vi "Main - Separate File and Output sessions.vi"() -> ()   [LabVIEW 2012]
uses:
  ChannelStateControl.ctl
  Imaging Pulse Control/Examples/Support/Channel Parameters.ctl
  Imaging Pulse Control/Examples/Support/System Parameters.ctl
  <vilib>/UeiDaq/UeiDaqCreateDOSession.vi
  <vilib>/UeiDaq/UeiDaqConfigureTimingForSimpleIO.vi
  <vilib>/UeiDaq/UeiDaqWriteDigitalDataUInt16.vi
  <vilib>/UeiDaq/UeiDaqWriteOneDigitalScanUInt16.vi
  <resource>/objmgr/UeiDaq.rc
  <vilib>/Utility/error.llb/DialogType.ctl
  <vilib>/ULx/Write.llb/ULx Write (Analog 1D DBL NChan 1Samp).vi
  Imaging Pulse Control/Quantum Composers 9000 Series.lvlib
  <vilib>/ULx/Create Channel.llb/ULx Create Channel (AO-Voltage-Basic).vi
  IPG Pulse Control/Agilent 33XXX Series.lvlib
  Agilent ESG Series/Agilent ESG Series.lvlib
panel:
  out "Timing Changed?":bool
  in  "Generate Form Switch":bool
  out "Period":dbl
  in  "#DIO Ports (Adjustable)":i32
  in  "Composer Write":bool
  in  "VISA session":refnum<visa-resource-name>
  in  "error in (no error)":errorcluster {"code" format="%.0x"}
  out "error out":errorcluster {"code" format="%.0x"}
  in  "Frequency (MHz)":dbl=224.0 format="%.11f"
  in  "Amplitude (dBm)":dbl=7.0 format="%.2f"
  in  "Output Enable":bool=TRUE
  out "Offset":dbl
  out "Amplitude":dbl
  in  "Maximum Voltage":dbl=10.0
  in  "Initial Voltage":dbl=2.0
  in  "Final Voltage":dbl=4.0
  out "Frequency":dbl=0.4838
  in  "Trigger Source (0: Internal)":u16(ring)=1 items=["Internal", "External", "Software (bus)"]
  in  "Enable Burst":bool=TRUE
  in  "Burst Mode (0: Triggered)":u16(ring) items=["Triggered", "Gated"]
  out "Simulated WaveForm":dbl[](graph)
  out "Total Time  (<16000)":i32
  in  "Final Keep Time":i32=100
  in  "Fall Down Time":i32=1000
  in  "Rise Up Time":i32=15
  in  "Pulse Width":i32=100
  in  "Inintial Voltage Time":i32=1
  in  "IPG Controller (Agilent 33210A)":refnum<visa-resource-name>
  in  "Arbitrary Waveform Name":string="ARB1"
  in  "Run IPG Laser  Switch":bool
  in  "Normal Stop":bool
  in  "Voltage (V)":dbl[](array[numeric])
  out "Initial States":u16[](array[numeric])
  in  "DIO Groups":T1[](array[typedef])=[{"Channel 1"=0, "Enable"=TRUE, "Main Switch"=0, "Channel 2"=0, "Channel 9"=0, "Channel 10"=0, "Channel 11"=0, "Channel 3"=0, "Channel 4"=0, "Channel 12"=0, "Channel 5"=0, "Channel 13"=0, "Channel 6"=0, "Channel 14"=0, "Channel 7"=0, "Channel 15"=0, "Channel 8"=0, "Channel 16"=0}, {"Channel 1"=0, "Enable"=TRUE, "Main Switch"=0, "Channel 2"=0, "Channel 9"=0, "Channel 10"=0, "Channel 11"=0, "Channel 3"=0, "Channel 4"=0, "Channel 12"=0, "Channel 5"=0, "Channel 13"=0, "Channel 6"=0, "Channel 14"=0, "Channel 7"=0, "Channel 15"=0, "Channel 8"=0, "Channel 16"=0}, {"Channel 1"=0, "Enable"=TRUE, "Main Switch"=0, "Channel 2"=0, "Channel 9"=0, "Channel 10"=0, "Channel 11"=0, "Channel 3"=0, "Channel 4"=0, "Channel 12"=0, "Channel 5"=0, "Channel 13"=0, "Channel 6"=0, "Channel 14"=0, "Channel 7"=0, "Channel 15"=0, "Channel 8"=0, "Channel 16"=0}, {"Channel 1"=0, "Enable"=TRUE, "Main Switch"=0, "Channel 2"=0, "Channel 9"=0, "Channel 10"=0, "Channel 11"=0, "Channel 3"=0, "Channel 4"=0, "Channel 12"=0, "Channel 5"=0, "Channel 13"=0, "Channel 6"=0, "Channel 14"=0, "Channel 7"=0, "Channel 15"=0, "Channel 8"=0, "Channel 16"=0}, {"Channel 1"=0, "Enable"=TRUE, "Main Switch"=0, "Channel 2"=0, "Channel 9"=0, "Channel 10"=0, "Channel 11"=0, "Channel 3"=0, "Channel 4"=0, "Channel 12"=0, "Channel 5"=0, "Channel 13"=0, "Channel 6"=0, "Channel 14"=0, "Channel 7"=0, "Channel 15"=0, "Channel 8"=0, "Channel 16"=0}, {"Channel 1"=0, "Enable"=TRUE, "Main Switch"=0, "Channel 2"=0, "Channel 9"=0, "Channel 10"=0, "Channel 11"=0, "Channel 3"=0, "Channel 4"=0, "Channel 12"=0, "Channel 5"=0, "Channel 13"=0, "Channel 6"=0, "Channel 14"=0, "Channel 7"=0, "Channel 15"=0, "Channel 8"=0, "Channel 16"=0}]
  out "Quantum Composer Command":string[](array[string])
  in  "Sys Period (s)":dbl=0.15
  out "Composer Ready?":bool
  out "Main Loop Stopped?":bool
  in  "Quantum Composer Resource":refnum<visa-resource-name>
  in  "Run/Stop":bool caption="stop"
  in  "Exit":bool
  out "Running 2":bool
  in  "Maximum Value":dbl=5.5 format="%0.2f"
  in  "Minimum Value":dbl format="%0.2f"
  out "Status Indicator":bool[][](array[boolean])
  out "Total Step":u64
  out "Original Timing Signal":i16[][](array[numeric]) format="%b"
  out "Running":bool
  in  "DIO Port":string="pwrdaq://Dev0/Do0:2"
  in  "stop":bool
  out "Loop Count":i32
  in  "Loop":bool
  out "Parsed File Location":path
  in  "All Low":bool
  in  "Run":bool
  in  "Timing Array (Adjustable)":i32[](array[numeric])=[0, 0, 0, 0, 0, 0, 0, 0, 0, 0, 0, 0, 0, 0, 0, 0, 0, 0, 0, 0] caption="Timing Array (Time Duration for each signal)"
  in  "Modified Timing Signal":i16[][](array[numeric])=[[0, 0, 0, 0, 0, 0, 0, 0, 0, 0, 0, 0, 0, 0, 0, 0, 0, 0, 0, 0]] caption="Modified Timing Signal (after adjustment from I/O channel panel)" format="%b"
  in  "Compile and Load":bool
  out "Channel Names":string[](array[string])
  out "Channel Number":u16=48
  in  "Timing File":path
  in  "Perl Parser":path=path "C:/Labview/Parser File/parse-timing.pl"
  # "MCCDAQ Control"
  # "Quantum Composer Control"
  # "(Use Do0:5 for DIO0-DIO5, 6ch,  Do0;5 for DIO0 and DIO5, 2ch)"
  # "Control Panel"
  # "(pwrdaq://Dev0 for real I/O; simu://Dev2 for simulated DAQ card)"
  # "1"
  # "2"
  # "3"
  # "4"
  # "5"
  # "6"
  # "7"
  # "8"
  # "9"
  # "10"
  # "11"
  # "12"
  # "13"
  # "14"
  # "15"
  # "16"
  # "Read me: (Very Important!!!!!!!!!)\n1. This Labview is used to control the IPG laser output power, When you edit this programme make sure the IPG laser is off.\n2. follow the steps, First is the visa address setting; Second is the pulse edit; Third is the output checking; Forth is the trigger set .\n3. The maximum input voltage is 10V, the minmum value is 1V. The total input time must smaller than 16000ms and larger than 8 ms."
  # "Group1"
  # "Group2"
  # "Group3"
  # "IPG Modulation Control"
  # "Offset Locking Control"
  # "Group4"
  # "Group5"
  # "Group6"
  # "(Currently, When \"STOP Loop\" is pressed, the status remain in the final state, when Stop Program or ER stop is pressed, all channels will be set as \"low\")"
  # "Status Panel"
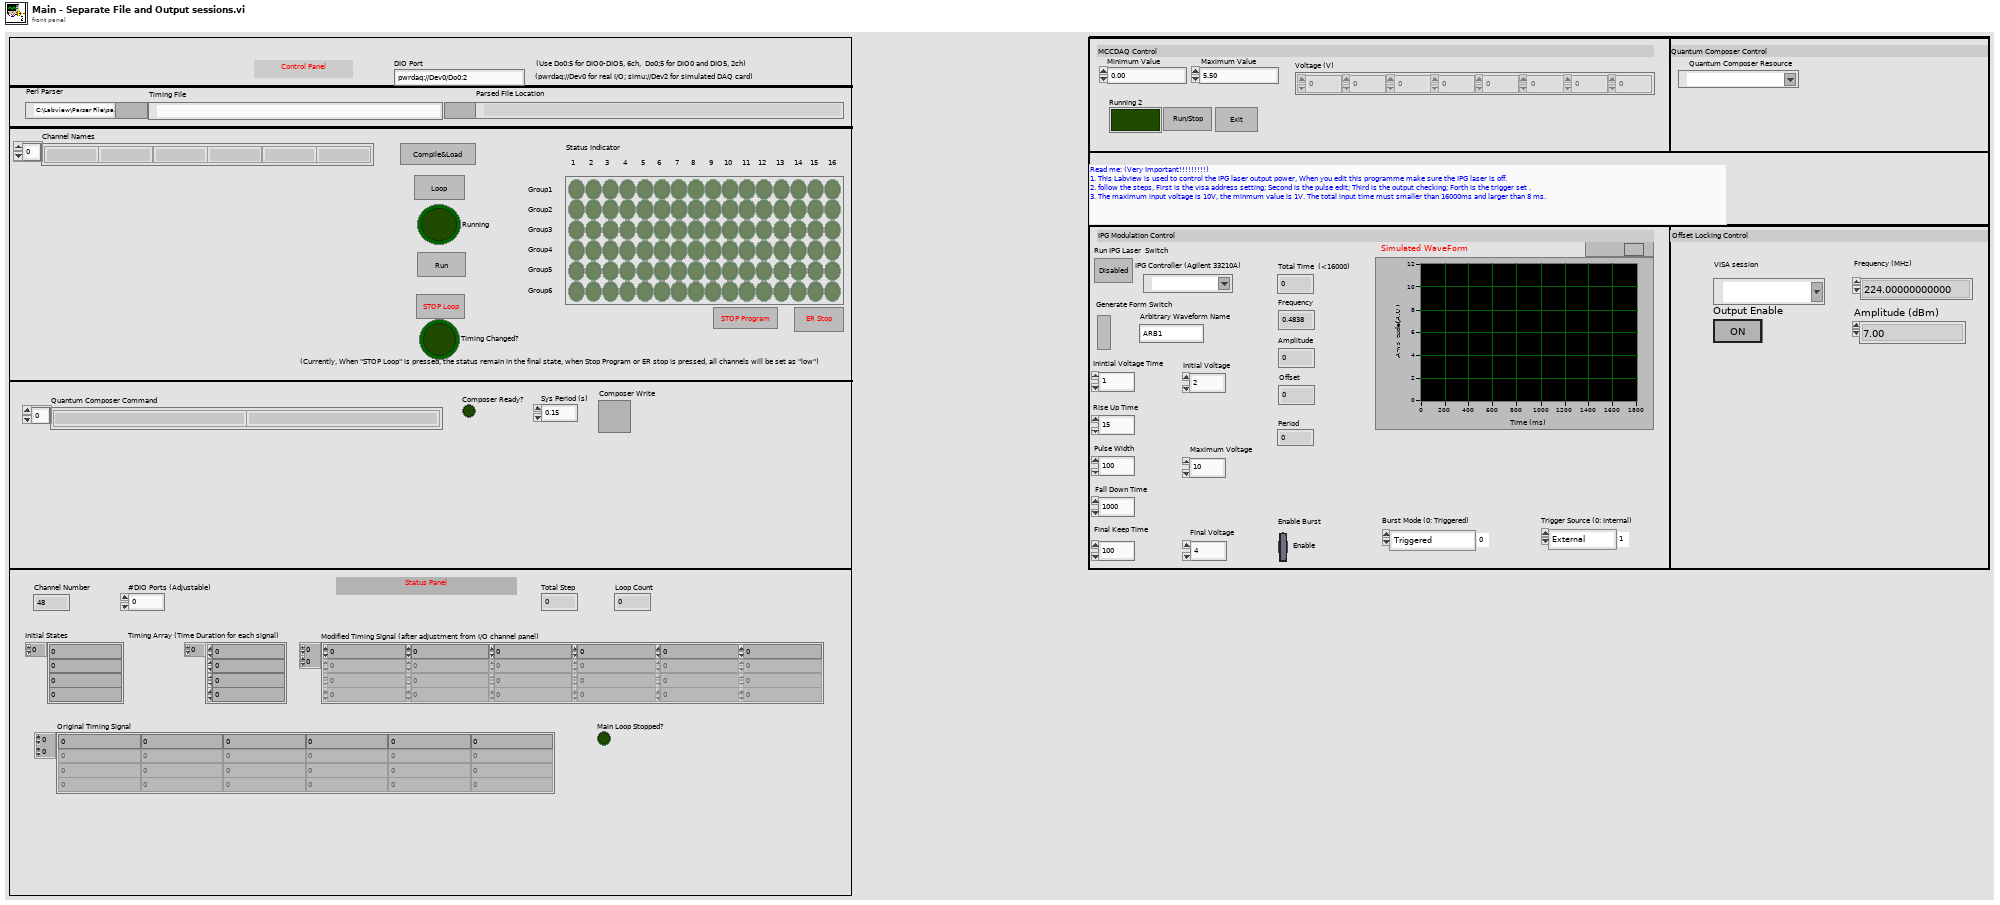
[diagram p1: front panel]
types:
  T1 = typedef "ChannelStateControl.ctl" = cluster{"Channel 1":u8, "Enable":bool, "Main Switch":u8, "Channel 2":u8, "Channel 9":u8, "Channel 10":u8, "Channel 11":u8, "Channel 3":u8, "Channel 4":u8, "Channel 12":u8, "Channel 5":u8, "Channel 13":u8, "Channel 6":u8, "Channel 14":u8, "Channel 7":u8, "Channel 15":u8, "Channel 8":u8, "Channel 16":u8}
  T2 = typedef "Channel Parameters.ctl" = cluster{"Channel":i32, "Chan State":bool, "Chan Sync Source":i32, "Chan Gate Logic":enum16{"Disabled", "Low", "High"}, "Chan Mode":enum16{"Normal", "Single", "Burst", "Duty Cycle"}, "Chan Wait #":i32, "Chan Delay":dbl, "Chan Width":dbl, "Chan Burst #":i32, "Chan DC On":i32, "Chan DC Off":i32, "Chan Polarity":bool, "Chan MUX Value":i32, "Chan Level Out":enum16{"TTL", "Adjustable", "35 Volt", "Optical"}, "Chan Lev Adjust":dbl, "Chan Gate Mode":enum16{"Disabled", "Pulse Inhibit", "Output Inhibit"}}
  T3 = enum16{"dBm", "dBuV", "dBuVemf", "mV", "uV", "mVemf", "uVemf"}
  T4 = enum16{"SINE", "TRIANGLE", "SQUARE", "RAMP", "NOISE", "DUAL SINE", "SWEPT SINE"}
  T5 = typedef "DialogType.ctl" = u16
  T6 = typedef "System Parameters.ctl" = cluster{"Sys Period":dbl, "Sys Mode":enum16{"Normal", "Single", "Burst", "Duty Cycle"}, "Sys Burst #":i32, "Sys DC On":i32, "Sys DC Off":i32, "Sys State":bool, "Sys Gate":bool, "Sys Trig Edge":bool, "Sys Ext Mode":enum16{"Disabled", "Triggered", "Gated", "Triggered & Gated"}, "Sys Trig Lev":dbl, "Sys Gate Lev ":dbl, "Sys Gate Mode":enum16{"Disabled", "Pulse Inhibit", "Output Inhibit", "Channel"}}
  T7 = cluster{"Baud Rate":u32, "Parity":u16, "Data Bits":u16, "Flow Control":u16}
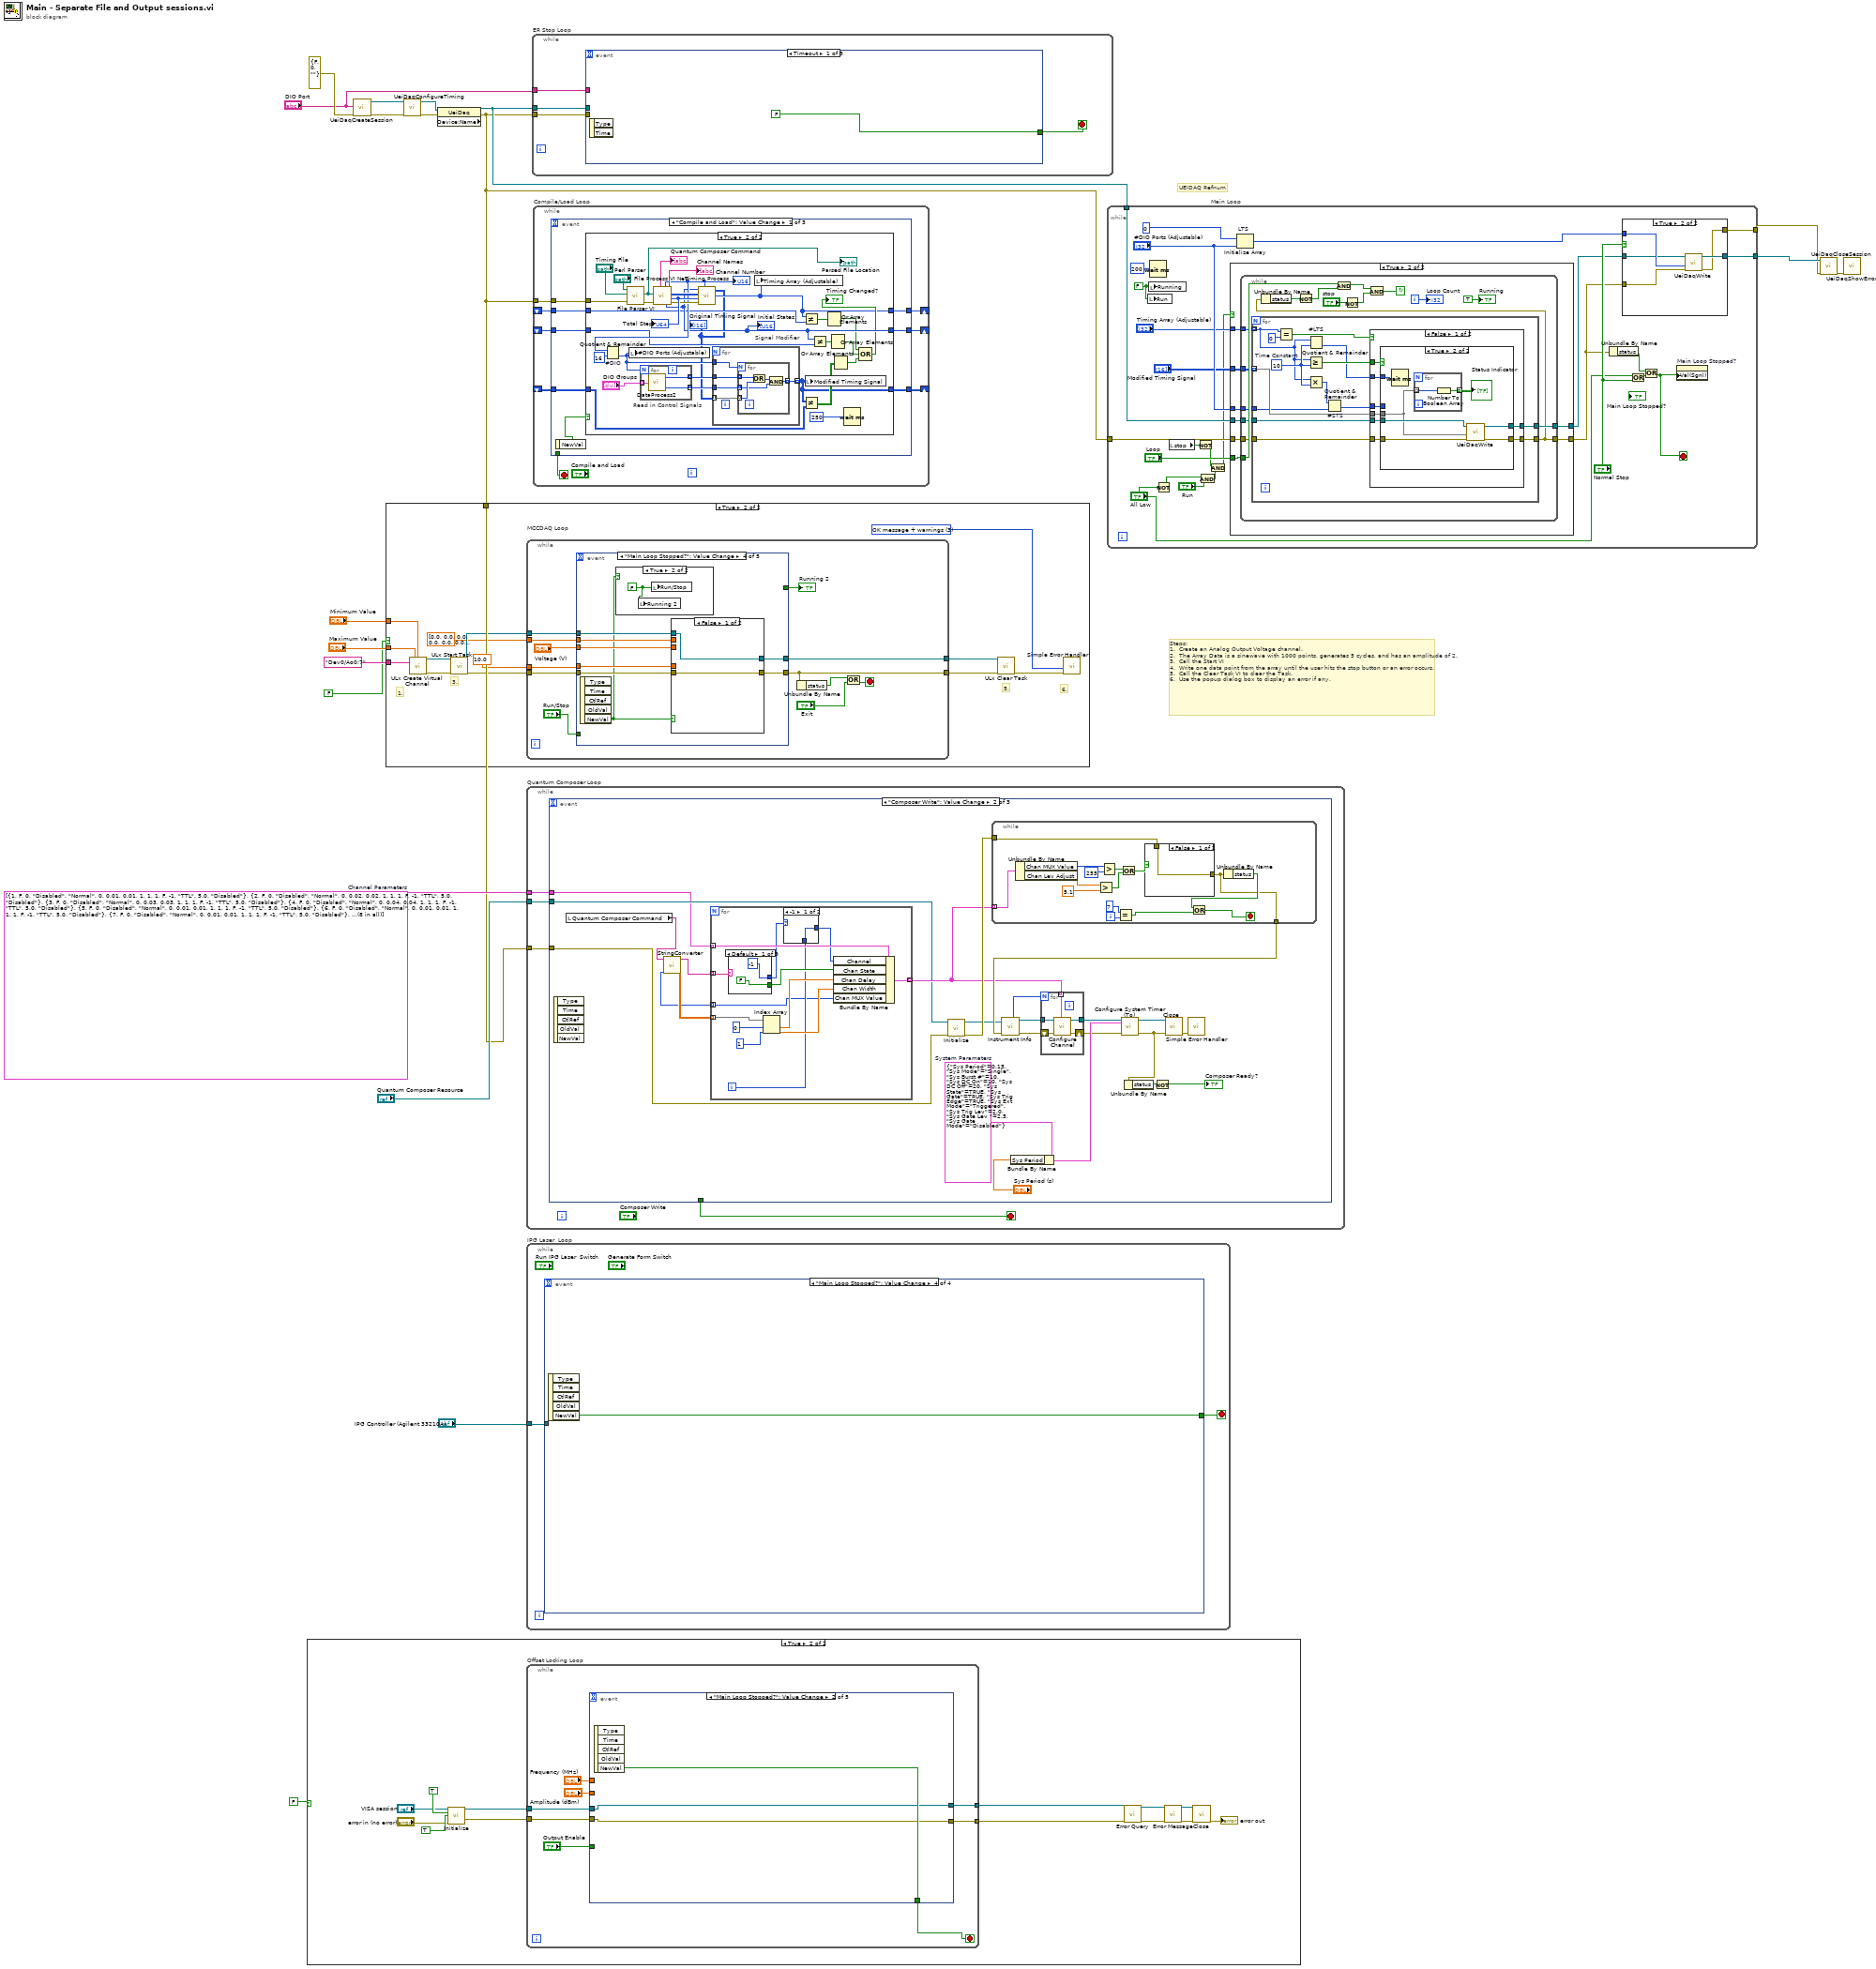
[diagram p0: block diagram]
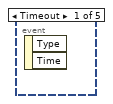
[diagram p3: hidden frame]
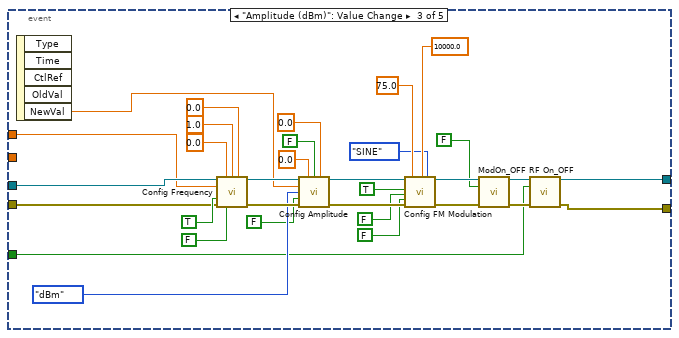
[diagram p4: hidden frame]
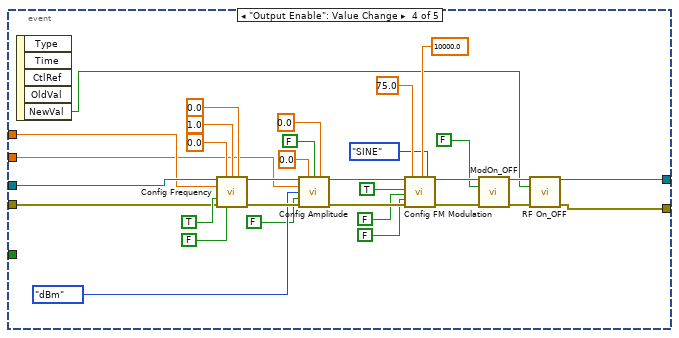
[diagram p5: hidden frame]
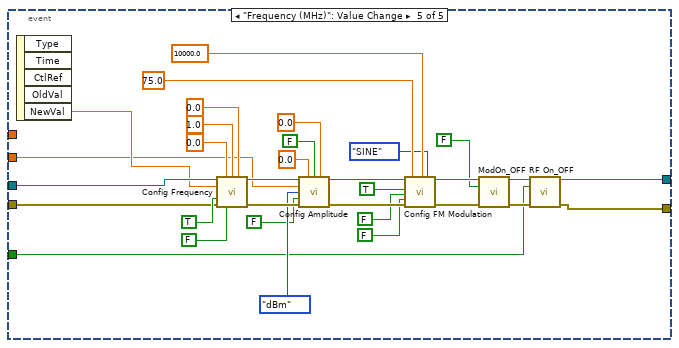
[diagram p6: hidden frame]
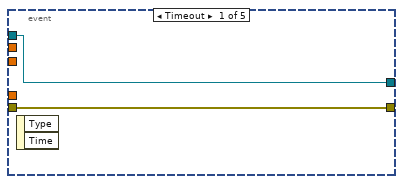
[diagram p8: hidden frame]
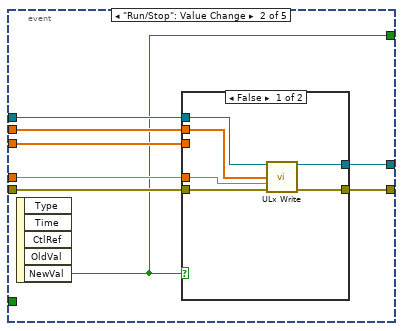
[diagram p9: hidden frame]
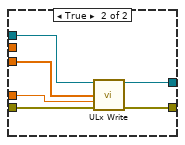
[diagram p10: hidden frame]
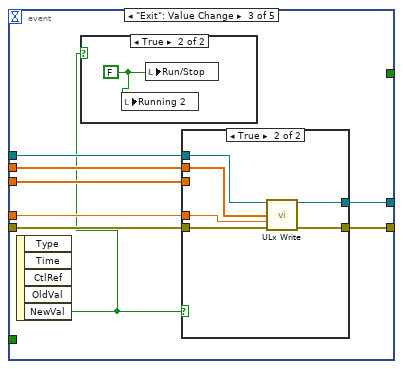
[diagram p11: hidden frame]
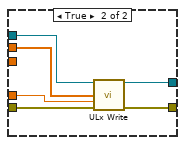
[diagram p15: hidden frame]
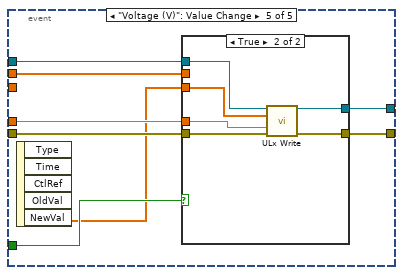
[diagram p16: hidden frame]
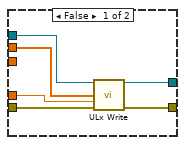
[diagram p17: hidden frame]
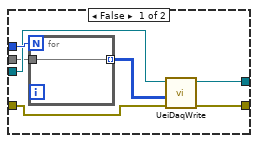
[diagram p20: hidden frame]
diagram:
  w8 = T2[] [{"Channel"=1, "Chan State"=FALSE, "Chan Sync Source"=0, "Chan Gate Logic"=enum."Disabled", "Chan Mode"=enum."Normal", "Chan Wait #"=0, "Chan Delay"=0.01, "Chan Width"=0.01, "Chan Burst #"=1, "Chan DC On"=1, "Chan DC Off"=1, "Chan Polarity"=FALSE, "Chan MUX Value"=-1, "Chan Level Out"=enum."TTL", "Chan Lev Adjust"=5.0, "Chan Gate Mode"=enum."Disabled"}, {"Channel"=2, "Chan State"=FALSE, "Chan Sync Source"=0, "Chan Gate Logic"=enum."Disabled", "Chan Mode"=enum."Normal", "Chan Wait #"=0, "Chan Delay"=0.02, "Chan Width"=0.02, "Chan Burst #"=1, "Chan DC On"=1, "Chan DC Off"=1, "Chan Polarity"=FALSE, "Chan MUX Value"=-1, "Chan Level Out"=enum."TTL", "Chan Lev Adjust"=5.0, "Chan Gate Mode"=enum."Disabled"}, {"Channel"=3, "Chan State"=FALSE, "Chan Sync Source"=0, "Chan Gate Logic"=enum."Disabled", "Chan Mode"=enum."Normal", "Chan Wait #"=0, "Chan Delay"=0.03, "Chan Width"=0.03, "Chan Burst #"=1, "Chan DC On"=1, "Chan DC Off"=1, "Chan Polarity"=FALSE, "Chan MUX Value"=-1, "Chan Level Out"=enum."TTL", "Chan Lev Adjust"=5.0, "Chan Gate Mode"=enum."Disabled"}, {"Channel"=4, "Chan State"=FALSE, "Chan Sync Source"=0, "Chan Gate Logic"=enum."Disabled", "Chan Mode"=enum."Normal", "Chan Wait #"=0, "Chan Delay"=0.04, "Chan Width"=0.04, "Chan Burst #"=1, "Chan DC On"=1, "Chan DC Off"=1, "Chan Polarity"=FALSE, "Chan MUX Value"=-1, "Chan Level Out"=enum."TTL", "Chan Lev Adjust"=5.0, "Chan Gate Mode"=enum."Disabled"}, {"Channel"=5, "Chan State"=FALSE, "Chan Sync Source"=0, "Chan Gate Logic"=enum."Disabled", "Chan Mode"=enum."Normal", "Chan Wait #"=0, "Chan Delay"=0.01, "Chan Width"=0.01, "Chan Burst #"=1, "Chan DC On"=1, "Chan DC Off"=1, "Chan Polarity"=FALSE, "Chan MUX Value"=-1, "Chan Level Out"=enum."TTL", "Chan Lev Adjust"=5.0, "Chan Gate Mode"=enum."Disabled"}, {"Channel"=6, "Chan State"=FALSE, "Chan Sync Source"=0, "Chan Gate Logic"=enum."Disabled", "Chan Mode"=enum."Normal", "Chan Wait #"=0, "Chan Delay"=0.01, "Chan Width"=0.01, "Chan Burst #"=1, "Chan DC On"=1, "Chan DC Off"=1, "Chan Polarity"=FALSE, "Chan MUX Value"=-1, "Chan Level Out"=enum."TTL", "Chan Lev Adjust"=5.0, "Chan Gate Mode"=enum."Disabled"}, {"Channel"=7, "Chan State"=FALSE, "Chan Sync Source"=0, "Chan Gate Logic"=enum."Disabled", "Chan Mode"=enum."Normal", "Chan Wait #"=0, "Chan Delay"=0.01, "Chan Width"=0.01, "Chan Burst #"=1, "Chan DC On"=1, "Chan DC Off"=1, "Chan Polarity"=FALSE, "Chan MUX Value"=-1, "Chan Level Out"=enum."TTL", "Chan Lev Adjust"=5.0, "Chan Gate Mode"=enum."Disabled"}, {"Channel"=8, "Chan State"=FALSE, "Chan Sync Source"=0, "Chan Gate Logic"=enum."Disabled", "Chan Mode"=enum."Normal", "Chan Wait #"=0, "Chan Delay"=0.01, "Chan Width"=0.01, "Chan Burst #"=1, "Chan DC On"=1, "Chan DC Off"=1, "Chan Polarity"=FALSE, "Chan MUX Value"=-1, "Chan Level Out"=enum."TTL", "Chan Lev Adjust"=5.0, "Chan Gate Mode"=enum."Disabled"}]  # Channel Parameters
  # "UEIDAQ Refnum"
  # "Steps: \n1.  Create an Analog Output Voltage channel.\n2.  The Array Data is a sinewave with 1000 points, generates 5 cycles, and has an amplitude of 2.\n3.  Call the Start VI\n4.  Write one data point from the array until the user hits the stop button or an error occurs. \n5.  Call the Clear Task VI to clear the Task.\n6.  Use the popup dialog box to display an error if any."
  n1 = case shown="True" FALSE {
    frame False {
    }
    frame True {
      n2 = call "Initialize.vi"("VISA Resource Name"="VISA session", "ID Query? (T: Yes)"=TRUE, "Reset? (T: Yes)"=TRUE, "error in (no error)"="error in (no error)") -> ("VISA Resource Name Out"=w22:refnum<visa-resource-name>, "error out"=w21:errorcluster)  [unwired: 10 in]
      n3 = while "Offset Locking Loop" {
        tunnel: [w40] -> w27
        tunnel: w22 -> [w39]
        tunnel: w21 -> [w38]
        tunnel: [w37] -> w20
        stop <- w35 stop-if-true
        n4 = event shown="[1] \"Main Loop Stopped?\": Value Change" {
          selector: _ -> [_ _ _ _ _]
          dyn-events: _ -> [_ _ _ _ _]
          timeout: _ -> [_ _ _ _ _]
          tunnel: [_ w41 w50 w82 w114] -> w40
          tunnel: w39 -> [_ w42 w49 w81 w113]
          tunnel: w38 -> [_ w41 w48 w80 w112]
          tunnel: "Output Enable" -> [_ _ w47 _ w109]
          tunnel: [_ w42 w46 w79 w108] -> w37
          tunnel: "Frequency (MHz)" -> [_ _ w44 w78 _]
          tunnel: [_ w43 _ _ _] -> w35
          tunnel: "Amplitude (dBm)" -> [_ _ _ w77 w110]
          event Timeout {
            n5 = event-data() -> ()  [unwired: 1 in, 2 out]
          }
          event "Main Loop Stopped?": Value Change {
            n6 = event-data() -> ("NewVal"=w43:bool)  [unwired: 1 in, 4 out]
          }
          event "Amplitude (dBm)": Value Change {
            n7 = event-data() -> ("NewVal"=w45:dbl)  [unwired: 1 in, 4 out]
            n8 = call "Config Frequency.vi"("VISA Resource Name"=w49, "Freq Offset (0.0)"=0.0, "Freq Multiplier (1.0)"=1.0, "Adjust Phase (0.0)"=0.0, "Frequency (1000.0)"=w44, "Freq Ref (T:ON)"=TRUE, "error in (no error)"=w48, "OptPhNoise (F:MD2 > 10khzOffset)"=FALSE) -> ("VISA Resource Name Out"=w75:refnum<visa-resource-name>, "error out"=w74:errorcluster)  [unwired: 6 in]
            n9 = call "Config Amplitude.vi"("VISA Resource Name"=w75, "Ampl Ref Set (0.00)"=0.0, "Ampl Ref (F:OFF)"=FALSE, "Ampl Offset (0.00)"=0.0, "Amplitude (-135.00)"=w45, "Unit (0:dBm)"=T3."dBm", "Atten Hold (F:OFF)"=FALSE, "error in (no error)"=w74) -> ("VISA Resource Name Out"=w73:refnum<visa-resource-name>, "error out"=w72:errorcluster)  [unwired: 6 in]
            n10 = call "Config FM Modulation.vi"("VISA Resource Name"=w73, "Status (T:ON)"=TRUE, "EXT Source Coupling (F:DC)"=FALSE, "FM Deviation Couple (F:OFF)"=FALSE, "error in (no error)"=w72, "FM Deviation (1.0)"=75.0 ("FM Deviation (75)"), "FM Rate (400.0)"=10000.0 ("FM Rate (10000)"), "FM Waveform (0:SINE)"=T4."SINE") -> ("VISA Resource Name Out"=w71:refnum<visa-resource-name>, "error out"=w70:errorcluster)  [unwired: 10 in]
            n11 = call "ModOn_OFF.vi"("VISA Resource Name"=w71, "Status (T:ON)"=FALSE, "error in (no error)"=w70) -> ("VISA Resource Name Out"=w69:refnum<visa-resource-name>, "error out"=w68:errorcluster)  [unwired: 11 in]
            n12 = call "RF On_OFF.vi"("VISA Resource Name"=w69, "Status (T:ON)"=w47, "error in (no error)"=w68) -> ("VISA Resource Name Out"=w46:refnum<visa-resource-name>, "error out"=w50:errorcluster)  [unwired: 11 in]
          }
          event "Output Enable": Value Change {
            n13 = event-data() -> ("NewVal"=w76:bool)  [unwired: 1 in, 4 out]
            n14 = call "Config Frequency.vi"("VISA Resource Name"=w81, "Freq Offset (0.0)"=0.0, "Freq Multiplier (1.0)"=1.0, "Adjust Phase (0.0)"=0.0, "Frequency (1000.0)"=w78, "Freq Ref (T:ON)"=TRUE, "error in (no error)"=w80, "OptPhNoise (F:MD2 > 10khzOffset)"=FALSE) -> ("VISA Resource Name Out"=w107:refnum<visa-resource-name>, "error out"=w106:errorcluster)  [unwired: 6 in]
            n15 = call "Config Amplitude.vi"("VISA Resource Name"=w107, "Ampl Ref Set (0.00)"=0.0, "Ampl Ref (F:OFF)"=FALSE, "Ampl Offset (0.00)"=0.0, "Amplitude (-135.00)"=w77, "Unit (0:dBm)"=T3."dBm", "Atten Hold (F:OFF)"=FALSE, "error in (no error)"=w106) -> ("VISA Resource Name Out"=w105:refnum<visa-resource-name>, "error out"=w104:errorcluster)  [unwired: 6 in]
            n16 = call "Config FM Modulation.vi"("VISA Resource Name"=w105, "Status (T:ON)"=TRUE, "EXT Source Coupling (F:DC)"=FALSE, "FM Deviation Couple (F:OFF)"=FALSE, "error in (no error)"=w104, "FM Deviation (1.0)"=75.0 ("FM Deviation (75)"), "FM Rate (400.0)"=10000.0 ("FM Rate (10000)"), "FM Waveform (0:SINE)"=T4."SINE") -> ("VISA Resource Name Out"=w103:refnum<visa-resource-name>, "error out"=w102:errorcluster)  [unwired: 10 in]
            n17 = call "ModOn_OFF.vi"("VISA Resource Name"=w103, "Status (T:ON)"=FALSE, "error in (no error)"=w102) -> ("VISA Resource Name Out"=w101:refnum<visa-resource-name>, "error out"=w100:errorcluster)  [unwired: 11 in]
            n18 = call "RF On_OFF.vi"("VISA Resource Name"=w101, "Status (T:ON)"=w76, "error in (no error)"=w100) -> ("VISA Resource Name Out"=w79:refnum<visa-resource-name>, "error out"=w82:errorcluster)  [unwired: 11 in]
          }
          event "Frequency (MHz)": Value Change {
            n19 = event-data() -> ("NewVal"=w111:dbl)  [unwired: 1 in, 4 out]
            n20 = call "Config Frequency.vi"("VISA Resource Name"=w113, "Freq Offset (0.0)"=0.0, "Freq Multiplier (1.0)"=1.0, "Adjust Phase (0.0)"=0.0, "Frequency (1000.0)"=w111, "Freq Ref (T:ON)"=TRUE, "error in (no error)"=w112, "OptPhNoise (F:MD2 > 10khzOffset)"=FALSE) -> ("VISA Resource Name Out"=w139:refnum<visa-resource-name>, "error out"=w138:errorcluster)  [unwired: 6 in]
            n21 = call "Config Amplitude.vi"("VISA Resource Name"=w139, "Ampl Ref Set (0.00)"=0.0, "Ampl Ref (F:OFF)"=FALSE, "Ampl Offset (0.00)"=0.0, "Amplitude (-135.00)"=w110, "Unit (0:dBm)"=T3."dBm", "Atten Hold (F:OFF)"=FALSE, "error in (no error)"=w138) -> ("VISA Resource Name Out"=w137:refnum<visa-resource-name>, "error out"=w136:errorcluster)  [unwired: 6 in]
            n22 = call "Config FM Modulation.vi"("VISA Resource Name"=w137, "Status (T:ON)"=TRUE, "EXT Source Coupling (F:DC)"=FALSE, "FM Deviation Couple (F:OFF)"=FALSE, "error in (no error)"=w136, "FM Deviation (1.0)"=75.0 ("FM Deviation (75)"), "FM Rate (400.0)"=10000.0 ("FM Rate (10000)"), "FM Waveform (0:SINE)"=T4."SINE") -> ("VISA Resource Name Out"=w135:refnum<visa-resource-name>, "error out"=w134:errorcluster)  [unwired: 10 in]
            n23 = call "ModOn_OFF.vi"("VISA Resource Name"=w135, "Status (T:ON)"=FALSE, "error in (no error)"=w134) -> ("VISA Resource Name Out"=w133:refnum<visa-resource-name>, "error out"=w132:errorcluster)  [unwired: 11 in]
            n24 = call "RF On_OFF.vi"("VISA Resource Name"=w133, "Status (T:ON)"=w109, "error in (no error)"=w132) -> ("VISA Resource Name Out"=w108:refnum<visa-resource-name>, "error out"=w114:errorcluster)  [unwired: 11 in]
          }
        }
      }
      n25 = call "Error Query.vi"("VISA Resource Name"=w20, "error in (no error)"=w27) -> ("VISA Resource Name Out"=w29:refnum<visa-resource-name>, "error out"=w32:errorcluster)  [unwired: 10 in, 2 out]
      n26 = call "Error Message.vi"("VISA Resource Name"=w29, "error in (no error)"=w32) -> ("VISA Resource Name Out"=w30:refnum<visa-resource-name>, "error out"=w31:errorcluster)  [unwired: 9 in, 3 out]
      n27 = call "Close.vi"("VISA Resource Name"=w30, "error in (no error)"=w31) -> ("error out"=→"error out":errorcluster)  [unwired: 13 in]
    }
  }
  n28 = call-poly <vilib>:"UeiDaqCreateSession.vi"("error in (no error)"=errorcluster {"status"=FALSE, "code"=0, "source"=""} ("error constant"), "Resource"="DIO Port") -> ("error out"=w18:errorcluster, "UeiDaq Refnum Out"=w19:refnum<k20>)  [unwired: 8 in]
  n29 = call-poly <vilib>:"UeiDaqConfigureTiming.vi"("error in (no error)"=w18, "UeiDaq Refnum In"=w19) -> ("error out"=w16:errorcluster, "UeiDaq Refnum Out"=w17:refnum<k20>)  [unwired: 8 in]
  n30 = property class="UeiDaq" props=["Device:Name"](reference=w17, error in=w16) -> (reference out=w7:refnum<k20>, error out=w6:errorcluster)  [unwired: 1 out]
  n31 = case shown="True" FALSE {
    tunnel: "Minimum Value" -> [_ w153]
    tunnel: "Maximum Value" -> [_ w152]
    tunnel: "Dev0/Ao0:7" -> [_ w145]
    tunnel: w6 -> [_ w140]
    frame False {
    }
    frame True {
      w148 = T5 3 items=["no dialog", "OK message", "continue or stop message", "OK message + warnings", "continue/stop + warnings"] ("type of dialog (OK msg:1)")
      # "6."
      # "5."
      # "3."
      # "1."
      n32 = call-poly <vilib>:"ULx Create Virtual Channel.vi"("maximum value"=w152, "minimum value"=w153, "physical channels"=w145, "error in"=w140) -> ("task out"=w147:refnum<k24>, "error out"=w146:errorcluster)  [unwired: 10 in]
      n33 = call <vilib>:"ULx Start Task.vi"("task in"=w147, "error in"=w146) -> ("task out"=w149:refnum<k24>, "error out"=w151:errorcluster)  [unwired: 12 in]
      n34 = while "MCCDAQ Loop" {
        tunnel: w151 -> [w164]
        tunnel: w149 -> [w165]
        tunnel: dbl[] [0.0, 0.0, 0.0, 0.0, 0.0, 0.0, 0.0, 0.0] -> [w161]
        tunnel: [w163] -> w144
        tunnel: [w160] -> w143
        tunnel: 10.0 ("timeout") -> [w162]
        stop <- w159 stop-if-true
        n35 = event shown="[3] \"Main Loop Stopped?\": Value Change" {
          selector: _ -> [_ _ _ _ _]
          dyn-events: _ -> [_ _ _ _ _]
          timeout: _ -> [_ _ _ _ _]
          tunnel: w165 -> [w167 w175 w195 w212 w229]
          tunnel: w164 -> [w166 w174 w194 w211 w228]
          tunnel: w162 -> [_ w173 w193 w210 w227]
          tunnel: "Voltage (V)" -> [_ w172 w192 w209 _]
          tunnel: [w167 w171 w191 w208 w226] -> w163
          tunnel: [w166 w170 w190 w207 w225] -> w160
          tunnel: w161 -> [_ w169 w189 w206 w224]
          tunnel: "Run/Stop" -> [_ _ _ _ w223]
          tunnel: [_ w168 _ _ _] -> w155
          event Timeout {
            n36 = event-data() -> ()  [unwired: 1 in, 2 out]
          }
          event "Run/Stop": Value Change {
            n37 = event-data() -> ("NewVal"=w168:bool)  [unwired: 1 in, 4 out]
            n38 = case shown="False" w168 {
              tunnel: w175 -> [w179 w187]
              tunnel: w174 -> [w178 w186]
              tunnel: w173 -> [w180 w185]
              tunnel: w172 -> [_ w184]
              tunnel: [w177 w183] -> w171
              tunnel: [w176 w182] -> w170
              tunnel: w169 -> [w181 _]
              frame False {
                n39 = call-poly <vilib>:"ULx Write.vi"("task in"=w179, "data"=w181, "timeout"=w180, "error in"=w178) -> ("task out"=w177:refnum<k24>, "error out"=w176:errorcluster)  [unwired: 9 in, 1 out]
              }
              frame True {
                n40 = call-poly <vilib>:"ULx Write.vi"("task in"=w187, "data"=w184, "timeout"=w185, "error in"=w186) -> ("task out"=w183:refnum<k24>, "error out"=w182:errorcluster)  [unwired: 9 in, 1 out]
              }
            }
          }
          event "Exit": Value Change {
            n41 = event-data() -> ("NewVal"=w188:bool)  [unwired: 1 in, 4 out]
            n42 = case shown="True" w188 {
              frame False {
              }
              frame True {
                w196 = FALSE
                n43 = local write "Running 2"(w196) -> ()
                n44 = local write "Run/Stop"(w196) -> ()
              }
            }
            n45 = case shown="True" w188 {
              tunnel: w195 -> [w198 w204]
              tunnel: w194 -> [w197 w203]
              tunnel: w193 -> [_ w202]
              tunnel: w192 -> [_ _]
              tunnel: [w198 w201] -> w191
              tunnel: [w197 w200] -> w190
              tunnel: w189 -> [_ w199]
              frame False {
              }
              frame True {
                n46 = call-poly <vilib>:"ULx Write.vi"("task in"=w204, "data"=w199, "timeout"=w202, "error in"=w203) -> ("task out"=w201:refnum<k24>, "error out"=w200:errorcluster)  [unwired: 9 in, 1 out]
              }
            }
          }
          event "Main Loop Stopped?": Value Change {
            n47 = event-data() -> ("NewVal"=w205:bool)  [unwired: 1 in, 4 out]
            n48 = case shown="True" w205 {
              frame False {
              }
              frame True {
                w213 = FALSE
                n49 = local write "Running 2"(w213) -> ()
                n50 = local write "Run/Stop"(w213) -> ()
              }
            }
            n51 = case shown="False" w205 {
              tunnel: w212 -> [w215 w221]
              tunnel: w211 -> [w214 w220]
              tunnel: w210 -> [_ w219]
              tunnel: w209 -> [_ _]
              tunnel: [w215 w218] -> w208
              tunnel: [w214 w217] -> w207
              tunnel: w206 -> [_ w216]
              frame False {
              }
              frame True {
                n52 = call-poly <vilib>:"ULx Write.vi"("task in"=w221, "data"=w216, "timeout"=w219, "error in"=w220) -> ("task out"=w218:refnum<k24>, "error out"=w217:errorcluster)  [unwired: 9 in, 1 out]
              }
            }
          }
          event "Voltage (V)": Value Change {
            n53 = event-data() -> ("NewVal"=w222:dbl[])  [unwired: 1 in, 4 out]
            n54 = case shown="True" w223 {
              tunnel: w229 -> [w233 w241]
              tunnel: w228 -> [w232 w240]
              tunnel: w227 -> [w234 w239]
              tunnel: w222 -> [_ w238]
              tunnel: [w231 w237] -> w226
              tunnel: [w230 w236] -> w225
              tunnel: w224 -> [w235 _]
              frame False {
                n55 = call-poly <vilib>:"ULx Write.vi"("task in"=w233, "data"=w235, "timeout"=w234, "error in"=w232) -> ("task out"=w231:refnum<k24>, "error out"=w230:errorcluster)  [unwired: 9 in, 1 out]
              }
              frame True {
                n56 = call-poly <vilib>:"ULx Write.vi"("task in"=w241, "data"=w238, "timeout"=w239, "error in"=w240) -> ("task out"=w237:refnum<k24>, "error out"=w236:errorcluster)  [unwired: 9 in, 1 out]
              }
            }
          }
        }
        "Running 2" <- w155
        n57 = Unbundle By Name(w160) -> ("status"=w158:bool)
        n58 = Or(x=w158, y="Exit") -> (x .or. y?=w159:bool)
      }
      n59 = call <vilib>:"ULx Clear Task.vi"("task in"=w144, "error in"=w143) -> ("error out"=w150:errorcluster)  [unwired: 13 in]
      n60 = call <vilib>:"Simple Error Handler.vi"("type of dialog (OK msg:1)"=w148, "error in (no error)"=w150) -> ()  [unwired: 3 in, 5 out]
    }
  }
  n61 = while "Quantum Composer Loop" {
    tunnel: "Quantum Composer Resource" -> [w244]
    tunnel: w6 -> [w245]
    tunnel: w8 -> [w242]
    stop <- w243 stop-if-true
    n62 = event shown="[1] \"Composer Write\": Value Change" {
      selector: _ -> [_ _ _]
      dyn-events: _ -> [_ _ _]
      timeout: _ -> [_ _ _]
      tunnel: w245 -> [_ w247 _]
      tunnel: w244 -> [_ w249 _]
      tunnel: w242 -> [_ w248 _]
      tunnel: [_ _ w325] -> w243
      event Timeout {
        n63 = event-data() -> ()  [unwired: 1 in, 2 out]
      }
      event "Composer Write": Value Change {
        w259 = T6 {"Sys Period"=0.15, "Sys Mode"=enum."Single", "Sys Burst #"=10, "Sys DC On"=10, "Sys DC Off"=20, "Sys State"=TRUE, "Sys Gate"=TRUE, "Sys Trig Edge"=TRUE, "Sys Ext Mode"=enum."Triggered", "Sys Trig Lev"=2.0, "Sys Gate Lev "=2.5, "Sys Gate Mode"=enum."Disabled"}  # System Paramaters
        n64 = event-data() -> ()  [unwired: 1 in, 5 out]
        n65 = local read "Quantum Composer Command"() -> (w246:string[])
        n66 = call "StringConverter.vi"("Composer Command"=w246) -> ("Internal Channel Delay and Width"=w265:dbl[][], "Internal Channel Name"=w266:string[], "Mux Value"=w264:i32[])  [unwired: 8 in]
        n67 = for {
          tunnel: w248 -> [w304] mode=indexing
          tunnel: w266 -> [w298] mode=indexing
          tunnel: w265 -> [w302] mode=indexing
          tunnel: [w293] -> w251 mode=indexing
          tunnel: w264 -> [w292] mode=indexing
          i -> [w294]
          n68 = case shown="Default" w298 {
            tunnel: [-1 0 1 2 3 4 5 6 7] -> w296
            tunnel: [FALSE TRUE TRUE TRUE TRUE TRUE TRUE TRUE TRUE] -> w297
            frame Default {
            }
            frame "A" {
            }
            frame "B" {
            }
            frame "C" {
            }
            frame "D" {
            }
            frame "E" {
            }
            frame "F" {
            }
            frame "G" {
            }
            frame "H" {
            }
          }
          n69 = Index Array(array=w302, index #1=0, index #2=1) -> (element #1=w303:dbl, element #2=w299:dbl)
          n70 = case shown="-1" w296 {
            selector: w296 -> [_ w306]
            tunnel: [w305 w306] -> w295
            tunnel: w294 -> [w305 _]
            frame -1 {
            }
            frame Default {
            }
          }
          n71 = Bundle By Name(cluster=w304, "Channel"=w295, "Chan State"=w297, "Chan Delay"=w303, "Chan Width"=w299, "Chan MUX Value"=w292) -> (w293:T2)
        }
        n72 = call "Initialize.vi"("error in (no error)"=w247, "VISA resource name"=w249) -> ("error out"=w262:errorcluster, "VISA resource name out"=w250:refnum<visa-resource-name>)  [unwired: 8 in]
        n73 = while {
          tunnel: w251 -> [w289] mode=indexing
          tunnel: [w275] -> w263
          tunnel: w262 -> [w276]
          i -> [w287]
          stop <- w277 stop-if-true
          n74 = Unbundle By Name(w289) -> ("Chan MUX Value"=w282:i32, "Chan Lev Adjust"=w285:dbl)
          n75 = Greater?(x=w285, y=5.1) -> (0:w283:bool)
          n76 = Greater?(x=w282, y=255) -> (0:w280:bool)
          n77 = Equal?(x=7, y=w287) -> (x = y?=w279:bool)
          n78 = Or(x=w280, y=w283) -> (x .or. y?=w284:bool)
          n79 = case shown="False" w284 {
            tunnel: [w290 errorcluster {"status"=TRUE, "code"=11000, "source"="Error in Range"} ("error constant")] -> w275
            tunnel: w276 -> [w290 _]
            frame False {
            }
            frame True {
            }
          }
          n80 = Unbundle By Name(w275) -> ("status"=w278:bool)
          n81 = Or(x=w278, y=w279) -> (x .or. y?=w277:bool)
        }
        n82 = call "Instrument Info.vi"("error in (no error)"=w263, "VISA resource name"=w250) -> ("error out"=w253:errorcluster, "VISA resource name out"=w252:refnum<visa-resource-name>, "Channels"=w254:i32)  [unwired: 6 in, 1 out]
        n83 = Bundle By Name(cluster=w259, "Sys Period"="Sys Period (s)") -> (w261:T6)
        n84 = for {
          N: w254 -> [_]
          tunnel: [w274] -> w255
          tunnel: w251 -> [w273] mode=indexing
          tunnel: w252 -> [w272]
          shift-right: [w271] -> w256
          shift-left: w253 -> [w270]
          n85 = call "Configure Channel.vi"("Chan Parameters"=w273, "error in (no error)"=w270, "VISA resource name"=w272) -> ("error out"=w271:errorcluster, "VISA resource name out"=w274:refnum<visa-resource-name>)  [unwired: 7 in]
        }
        n86 = call "Configure System Timer (To).vi"("System Parameters"=w261, "error in (no error)"=w256, "VISA resource name"=w255) -> ("error out"=w269:errorcluster, "VISA resource name out"=w268:refnum<visa-resource-name>)  [unwired: 7 in]
        n87 = Unbundle By Name(w269) -> ("status"=w257:bool)
        n88 = Not(x=w257) -> (.not. x?=→"Composer Ready?":bool)
        n89 = call "Close.vi"("error in (no error)"=w269, "VISA resource name"=w268) -> ("error out"=w267:errorcluster)  [unwired: 9 in]
        n90 = call <vilib>:"Simple Error Handler.vi"("error in (no error)"=w267) -> ()  [unwired: 4 in, 5 out]
      }
      event "Main Loop Stopped?": Value Change {
        n91 = event-data() -> ("NewVal"=w325:bool)  [unwired: 1 in, 3 out]
      }
    }
  }
  n92 = while "IPG Laser  Loop" {
    tunnel: "IPG Controller (Agilent 33210A)" -> [w326]
    stop <- w327 stop-if-true
    n93 = event shown="[3] \"Main Loop Stopped?\": Value Change" {
      selector: _ -> [_ _ _ _]
      dyn-events: _ -> [_ _ _ _]
      timeout: _ -> [_ _ _ _]
      tunnel: [_ _ _ w409] -> w327
      tunnel: w326 -> [_ _ w385 _]
      event Timeout {
        n94 = event-data() -> ()  [unwired: 1 in, 2 out]
      }
      event "Generate Form Switch": Value Change {
        n95 = event-data() -> ()  [unwired: 1 in, 5 out]
        n96 = Subtract(x="Maximum Voltage", y="Final Voltage") -> (x-y=w339:dbl)
        n97 = Less?(x="Final Voltage", y="Initial Voltage") -> (x < y?=w338:bool)
        n98 = Subtract(x="Maximum Voltage", y="Initial Voltage") -> (x-y=w341:dbl)
        n99 = Select "Vmin"(t="Final Voltage", s=w338, f="Initial Voltage") -> (s? t:f=w334:dbl)
        n100 = Subtract(x="Maximum Voltage", y=w334) -> (x-y=w337:dbl)
        n101 = Divide(x=w337, y=2) -> (x/y=→"Amplitude":dbl)
        n102 = Add(x="Maximum Voltage", y=w334) -> (x+y=w333:dbl)
        n103 = Divide(x=w333, y=4) -> (x/y=→"Offset":dbl)
        n104 = for {
          N: "Fall Down Time" -> [w362]
          tunnel: [w367] -> w351 mode=indexing
          tunnel: w339 -> [w364]
          tunnel: "Maximum Voltage" -> [w363]
          i -> [w366]
          n105 = Increment(x=w366) -> (x+1=w365:i32)
          n106 = Multiply(x=w364, y=w365) -> (x*y=w369:dbl)
          n107 = Divide(x=w369, y=w362) -> (x/y=w368:dbl)
          n108 = Subtract(x=w363, y=w368) -> (x-y=w367:dbl)
        }
        n109 = for {
          N: "Rise Up Time" -> [w372]
          tunnel: [w377] -> w355 mode=indexing
          tunnel: "Initial Voltage" -> [w376]
          tunnel: w341 -> [w374]
          i -> [w378]
          n110 = Increment(x=w378) -> (x+1=w375:i32)
          n111 = Multiply(x=w374, y=w375) -> (x*y=w373:dbl)
          n112 = Divide(x=w373, y=w372) -> (x/y=w371:dbl)
          n113 = Add(x=w376, y=w371) -> (x+y=w377:dbl)
        }
        n114 = for {
          N: "Pulse Width" -> [_]
          tunnel: [w370] -> w352 mode=indexing
          tunnel: "Maximum Voltage" -> [w370]
        }
        n115 = for {
          N: "Final Keep Time" -> [_]
          tunnel: [w359] -> w349 mode=indexing
          tunnel: "Final Voltage" -> [w360]
          n116 = To Double Precision Float(number=w360) -> (double precision float=w359:dbl)
        }
        n117 = for {
          N: "Inintial Voltage Time" -> [_]
          tunnel: [w361] -> w353 mode=indexing
          tunnel: "Initial Voltage" -> [w361]
        }
        n118 = Insert Into Array(array=w353, new element #1=w355, new element #2=w352, new element #3=w351, new element #4=w349) -> (w342:dbl[])  [unwired: 1 in]
        "Simulated WaveForm" <- w342
        n119 = Array Size(array=w342) -> (size(s)=w346:i32)
        "Total Time  (<16000)" <- w346
        n120 = Divide(x=1000, y=w346) -> (x/y=→"Frequency":dbl)
        n121 = Divide(x=w346, y=1000) -> (x/y=w344:dbl)
        n122 = Add(x=0.1, y=w344) -> (x+y=→"Period":dbl)
      }
      event "Run IPG Laser  Switch": Value Change {
        w403 = u16 0 items=["Positive", "Negative"] ("Slope (0: Positive)")
        w387 = u32 30001  # Timeout (30000)
        (unwired) TRUE  # Enable Output (T: Enable)
        # "For large waveform transfers, increase the timeout value."
        n123 = event-data() -> ("NewVal"=w379:bool)  [unwired: 1 in, 4 out]
        n124 = local read "Simulated WaveForm"() -> (w381:dbl[])
        n125 = call "Initialize.vi"("Serial Configuration"=T7 {"Baud Rate"=9600, "Parity"=0, "Data Bits"=8, "Flow Control"=4}, "VISA resource name"=w385) -> ("error out"=w389:errorcluster, "VISA resource name out"=w391:refnum<visa-resource-name>)  [unwired: 8 in]
        n126 = call "Create Arbitrary Waveform.vi"("Timeout (10000)"=w387, "error in (no error)"=w389, "Arbitrary Waveform Data"=w381, "Arbitrary Waveform Name (\"ARB1\")"="Arbitrary Waveform Name", "VISA resource name"=w391) -> ("error out"=w388:errorcluster, "VISA resource name out"=w390:refnum<visa-resource-name>)  [unwired: 5 in]
        n127 = local read "Frequency"() -> (w382:dbl)
        n128 = local read "Amplitude"() -> (w384:dbl)
        n129 = local read "Offset"() -> (w383:dbl)
        n130 = call "Configure Arbitrary Waveform.vi"("Frequency (1000 Hz)"=w382, "Offset (0.00 V)"=w383, "error in (no error)"=w388, "Gain (1.0)"=w384, "Arbitrary Waveform Name (\"ARB1\")"="Arbitrary Waveform Name", "VISA resource name"=w390) -> ("error out"=w401:errorcluster, "VISA resource name out"=w402:refnum<visa-resource-name>)  [unwired: 4 in]
        n131 = call "Configure Trigger.vi"("Delay (0.0 s)"=0.0, "error in (no error)"=w401, "Slope (0: Positive)"=w403, "Trigger Source (0: Internal)"="Trigger Source (0: Internal)", "VISA resource name"=w402) -> ("error out"=w399:errorcluster, "VISA resource name out"=w400:refnum<visa-resource-name>)  [unwired: 5 in]
        n132 = local read "Period"() -> (w380:dbl)
        n133 = call "Configure Modulation (Burst).vi"("VISA resource name"=w400, "Burst Phase (0 deg)"=0, "Burst Count (1)"=1, "Burst Period (1 s)"=w380, "Enable Burst Modulation (T: Enable)"="Enable Burst", "Burst Modulation Mode (0: Triggered)"="Burst Mode (0: Triggered)", "error in (no error)"=w399) -> ("VISA resource name out"=w398:refnum<visa-resource-name>, "error out"=w397:errorcluster)  [unwired: 7 in]
        n134 = call "Enable Output.vi"("error in (no error)"=w397, "Enable Output  (T: Enable)"=w379, "VISA resource name"=w398) -> ("error out"=w407:errorcluster, "VISA resource name out"=w406:refnum<visa-resource-name>)  [unwired: 7 in]
        n135 = call "Close.vi"("error in (no error)"=w407, "VISA resource name"=w406) -> ("error out"=w408:errorcluster)  [unwired: 9 in]
        n136 = call <vilib>:"Simple Error Handler.vi"("error in (no error)"=w408) -> ()  [unwired: 4 in, 5 out]
      }
      event "Main Loop Stopped?": Value Change {
        n137 = event-data() -> ("NewVal"=w409:bool)  [unwired: 1 in, 4 out]
      }
    }
  }
  n138 = while "ER Stop Loop" {
    tunnel: w6 -> [w412]
    tunnel: w7 -> [w411]
    tunnel: "DIO Port" -> [w410]
    stop <- w413 stop-if-true
    n139 = event shown="[0] Timeout" {
      selector: _ -> [_ _ _]
      dyn-events: _ -> [_ _ _]
      timeout: _ -> [_ _ _]
      tunnel: [FALSE w431 w434] -> w413
      tunnel: w412 -> [_ w429 _]
      tunnel: w411 -> [_ w430 _]
      tunnel: w410 -> [_ w415 _]
      event Timeout {
        n140 = event-data() -> ()  [unwired: 1 in, 2 out]
      }
      event "All Low": Value Change {
        w420 = 8  # ALL State cleared regardless of status
        n141 = event-data() -> ("NewVal"=w431:bool)  [unwired: 1 in, 1 out]
        n142 = call <vilib>:"UeiDaqCloseSession.vi"("error in (no error)"=w429, "UeiDaq Refnum In"=w430) -> ("error out"=w416:errorcluster)  [unwired: 8 in, 1 out]
        n143 = local write "Running"(FALSE) -> ()
        n144 = call <vilib>:"UeiDaqShowError.vi"("error in (no error)"=w416) -> ()  [unwired: 10 in, 1 out]
        n145 = call-poly <vilib>:"UeiDaqCreateSession.vi"("error in (no error)"=w416, "Resource"=w415) -> ("error out"=w423:errorcluster, "UeiDaq Refnum Out"=w422:refnum<k20>)  [unwired: 8 in]
        n146 = Initialize Array "LTS"(i16 0, w420) -> (w421:i16[])
        n147 = call-poly <vilib>:"UeiDaqConfigureTiming.vi"("error in (no error)"=w423, "UeiDaq Refnum In"=w422) -> ("error out"=w425:errorcluster, "UeiDaq Refnum Out"=w424:refnum<k20>)  [unwired: 8 in]
        n148 = call-poly <vilib>:"UeiDaqWrite.vi"("error in (no error)"=w425, "Digital Data"=w421, "UeiDaq Refnum In"=w424) -> ("error out"=w418:errorcluster, "UeiDaq Refnum Out"=w417:refnum<k20>)  [unwired: 7 in]
        n149 = call <vilib>:"UeiDaqCloseSession.vi"("error in (no error)"=w418, "UeiDaq Refnum In"=w417) -> ("error out"=w427:errorcluster)  [unwired: 8 in, 1 out]
        n150 = flat-sequence {
          tunnel: [w433] -> w426
          tunnel: w427 -> [w433]
          frame #0 {
            w432 = FALSE
            n151 = local write "Loop"(w432) -> ()
            n152 = local write "Running"(w432) -> ()
            n153 = local write "All Low"(w432) -> ()
            n154 = local write "Run"(w432) -> ()
          }
        }
        n155 = call <vilib>:"UeiDaqShowError.vi"("error in (no error)"=w426) -> ()  [unwired: 10 in, 1 out]
      }
      event "Normal Stop": Value Change {
        n156 = event-data() -> ("NewVal"=w434:bool)  [unwired: 1 in, 3 out]
      }
    }
  }
  n157 = while "Compile/Load Loop" {
    tunnel: w6 -> [w442]
    shift-right: [w440] -> _
    shift-left: _ -> [w437]
    shift-right: [w439] -> _
    shift-left: _ -> [w435]
    shift-right: [w438] -> _
    shift-left: _ -> [w436]
    stop <- w441 stop-if-true
    n158 = event shown="[0] \"Compile and Load\": Value Change" {
      selector: _ -> [_ _ _]
      dyn-events: _ -> [_ _ _]
      timeout: _ -> [_ _ _]
      tunnel: w442 -> [w450 _ _]
      tunnel: [_ w501 _] -> w441
      tunnel: [w448 w500 w504] -> w440
      tunnel: [w447 w498 w502] -> w439
      tunnel: [w446 w499 w503] -> w438
      tunnel: w437 -> [w445 w500 w504]
      tunnel: w436 -> [w444 w499 w503]
      tunnel: w435 -> [w443 w498 w502]
      event "Compile and Load": Value Change {
        n159 = event-data() -> ("NewVal"=w449:bool)  [unwired: 1 in]
        n160 = case shown="True" w449 {
          tunnel: w450 -> [_ w473]
          tunnel: [w453 w456] -> w448
          tunnel: [w451 w463] -> w447
          tunnel: [w452 w466] -> w446
          tunnel: w445 -> [w453 w455]
          tunnel: w444 -> [w452 w465]
          tunnel: w443 -> [w451 w462]
          frame False {
          }
          frame True {
            n161 = call "File Parser VI.vi"("error in (no error)"=w473, "Original Timing File Path"="Timing File", "Perl Parser Path"="Perl Parser") -> ("error out"=w482:errorcluster, "Parsed File Path"=w480:path)  [unwired: 7 in]
            "Parsed File Location" <- w480
            n162 = call "File Process VI New.vi"("error in (no error)"=w482, "Parsed File Path"=w480) -> ("Error Out"=w472:errorcluster, "Total Step"=w478:u64, "Switching Times"=w479:u32[][], "Channel Names"=→"Channel Names":string[], "Initial States"=w466:u16[], "Channel Number"=w470:u16, "GPIB Output"=→"Quantum Composer Command":string[])  [unwired: 3 in]
            "Channel Number" <- w470
            "Total Step" <- w478
            "Initial States" <- w466
            n163 = Quotient & Remainder "#DIO"(x=w470, y=u16 16) -> (floor(x/y)=w457:u16)  [unwired: 1 out]
            n164 = local write "#DIO Ports (Adjustable)"(w457) -> ()
            n165 = for "Read in Control Signals" {
              N: w457 -> [_]
              tunnel: "DIO Groups" -> [w487] mode=indexing
              tunnel: [w486] -> w476 mode=indexing
              tunnel: [w485] -> w475 mode=indexing
              n166 = call "DataProcess2.vi"("DIO Group 1"=w487) -> ("High"=w486:u16, "Low"=w485:u16)
            }
            n167 = call "Timing Process.vi"("Initial States"=w466, "Switching Times"=w479, "Total Steps"=w478, "error in (no error)"=w472, "Channel"=w470) -> ("Output Signal Array"=w454:i16[][], "Output Time Array"=w456:i32[])  [unwired: 1 out]
            "Original Timing Signal" <- w454
            n168 = for "Signal Modifier" {
              tunnel: w454 -> [w492] mode=indexing
              tunnel: [w491] -> w463 mode=indexing
              tunnel: w476 -> [w490]
              tunnel: w475 -> [w489]
              tunnel: w457 -> [w488]
              n169 = for {
                N: w488 -> [_]
                tunnel: w492 -> [w497] mode=indexing
                tunnel: [w495] -> w491 mode=indexing
                tunnel: w490 -> [w494] mode=indexing
                tunnel: w489 -> [w493] mode=indexing
                n170 = Or(x=w494, y=w497) -> (x .or. y?=w496:u16)
                n171 = And(x=w496, y=w493) -> (x .and. y?=w495:u16)
              }
            }
            n172 = local write "Timing Array (Adjustable)"(w456) -> ()
            n173 = Not Equal?(x=w456, y=w455) -> (x != y?=w468:bool[])
            n174 = Not Equal?(x=w463, y=w462) -> (x != y?=w464:bool[][])
            n175 = local write "Modified Timing Signal"(w463) -> ()
            n176 = Not Equal?(x=w466, y=w465) -> (x != y?=w467:bool[])
            n177 = Or Array Elements(Boolean array=w468) -> (logical OR=w461:bool)
            n178 = Or Array Elements(Boolean array=w467) -> (logical OR=w460:bool)
            n179 = Or Array Elements(Boolean array=w464) -> (logical OR=w459:bool)
            n180 = Wait (ms)(milliseconds to wait=250) -> ()  [unwired: 1 out]
            n181 = Compound Arithmetic op=OR(w461, w460, w459) -> (→"Timing Changed?":bool)
          }
        }
      }
      event "Main Loop Stopped?": Value Change {
        n182 = event-data() -> ("NewVal"=w501:bool)  [unwired: 1 in]
      }
      event Timeout {
        n183 = event-data() -> ()  [unwired: 1 in, 2 out]
      }
    }
  }
  n184 = while "Main Loop" {
    tunnel: w7 -> [w516]
    tunnel: w6 -> [w514]
    tunnel: [w512] -> w5
    tunnel: [w511] -> w4
    stop <- w515 stop-if-true
    w518 = FALSE
    n185 = local write "Run"(w518) -> ()
    n186 = local write "Running"(w518) -> ()
    n187 = Wait (ms)(milliseconds to wait=200) -> ()  [unwired: 1 out]
    n188 = Not(x="All Low") -> (.not. x?=w527:bool)
    n189 = local read "stop"() -> (w506:bool)
    n190 = Not(x=w506) -> (.not. x?=w505:bool)
    n191 = And(x=w527, y="Run") -> (x .and. y?=w508:bool)
    n192 = And(x=w505, y=w508) -> (x .and. y?=w507:bool)
    n193 = case shown="True" w507 {
      tunnel: "Loop" -> [_ w546]
      tunnel: [w537 w545] -> w524
      tunnel: [w538 w544] -> w523
      tunnel: w516 -> [w538 w543]
      tunnel: w514 -> [w537 w542]
      tunnel: "Timing Array (Adjustable)" -> [_ w541]
      tunnel: "Modified Timing Signal" -> [_ w540]
      tunnel: "#DIO Ports (Adjustable)" -> [_ w539]
      frame False {
      }
      frame True {
        n194 = while {
          tunnel: w546 -> [w555]
          tunnel: [w556] -> w545
          tunnel: [w562] -> w544
          tunnel: w543 -> [w551]
          tunnel: w542 -> [w550]
          tunnel: w541 -> [w549]
          tunnel: w540 -> [w548]
          tunnel: w539 -> [w547]
          i -> [w561]
          stop <- w559 continue-if-true
          n195 = for {
            tunnel: [w575] -> w556
            tunnel: [w573] -> w562
            tunnel: w551 -> [w567]
            tunnel: w550 -> [w566]
            tunnel: w549 -> [w563] mode=indexing
            tunnel: w548 -> [w565] mode=indexing
            tunnel: w547 -> [w564]
            w568 = 10  # Time Constant
            n196 = Equal?(x=w563, y=0) -> (x = y?=w571:bool)
            n197 = Greater Or Equal?(x=w563, y=w568) -> (x >= y?=w576:bool)
            n198 = Multiply(x=w563, y=w568) -> (x*y=w570:i32)
            n199 = Quotient & Remainder "#LTS"(x=w563, y=w568) -> (floor(x/y)=w574:i32)  [unwired: 1 out]
            n200 = Quotient & Remainder "#STS"(x=w570, y=w564) -> (floor(x/y)=w569:i32)  [unwired: 1 out]
            n201 = case shown="False" w571 {
              tunnel: w576 -> [w584 _]
              tunnel: [w583 w602] -> w575
              tunnel: w574 -> [w582 _]
              tunnel: [w581 w603] -> w573
              tunnel: w569 -> [w580 _]
              tunnel: w567 -> [w579 w603]
              tunnel: w566 -> [w578 w602]
              tunnel: w565 -> [w577 _]
              frame False {
                n202 = case shown="True" w584 {
                  tunnel: [w591 w599] -> w583
                  tunnel: w582 -> [_ w598]
                  tunnel: [w590 w597] -> w581
                  tunnel: w580 -> [w589 _]
                  tunnel: w579 -> [w588 w595]
                  tunnel: w578 -> [w587 w594]
                  tunnel: w577 -> [w585 w593]
                  frame False {
                    n203 = for {
                      N: w589 -> [_]
                      tunnel: [w592] -> w586 mode=indexing
                      tunnel: w585 -> [w592]
                    }
                    n204 = call-poly <vilib>:"UeiDaqWrite.vi"("error in (no error)"=w587, "Digital Data"=w586, "UeiDaq Refnum In"=w588) -> ("error out"=w591:errorcluster, "UeiDaq Refnum Out"=w590:refnum<k20>)  [unwired: 7 in]
                  }
                  frame True {
                    n205 = Wait (ms)(milliseconds to wait=w598) -> ()  [unwired: 1 out]
                    n206 = for {
                      tunnel: [w601] -> w596 mode=indexing
                      tunnel: w593 -> [w600] mode=indexing
                      n207 = Number To Boolean Array(number=w600) -> (Boolean array=w601:bool[])
                    }
                    "Status Indicator" <- w596
                    n208 = call-poly <vilib>:"UeiDaqWrite.vi"("error in (no error)"=w594, "Digital Data"=w593, "UeiDaq Refnum In"=w595) -> ("error out"=w599:errorcluster, "UeiDaq Refnum Out"=w597:refnum<k20>)  [unwired: 7 in]
                  }
                }
              }
              frame True {
              }
            }
          }
          n209 = Unbundle By Name(w556) -> ("status"=w557:bool)
          n210 = Not(x=w557) -> (.not. x?=w554:bool)
          n211 = And(x=w555, y=w554) -> (x .and. y?=w553:bool)
          n212 = Not(x="stop") -> (.not. x?=w552:bool)
          n213 = And(x=w553, y=w552) -> (x .and. y?=w559:bool)
          "Loop Count" <- w561
          "Running" <- TRUE
        }
      }
    }
    n214 = Initialize Array "LTS"(i16 0, "#DIO Ports (Adjustable)") -> (w522:i16[])
    n215 = Unbundle By Name(w524) -> ("status"=w520:bool)
    n216 = case shown="True" "Normal Stop" {
      tunnel: w522 -> [_ w536]
      tunnel: w523 -> [w531 w535]
      tunnel: [w531 w534] -> w512
      tunnel: w524 -> [w530 w533]
      tunnel: [w530 w532] -> w511
      frame False {
      }
      frame True {
        n217 = call-poly <vilib>:"UeiDaqWrite.vi"("error in (no error)"=w533, "Digital Data"=w536, "UeiDaq Refnum In"=w535) -> ("error out"=w532:errorcluster, "UeiDaq Refnum Out"=w534:refnum<k20>)  [unwired: 7 in]
      }
    }
    n218 = Or(x="All Low", y="Normal Stop") -> (x .or. y?=w528:bool)
    n219 = Or(x=w520, y=w528) -> (x .or. y?=w515:bool)
    n220 = property on="Main Loop Stopped?" class="Bool (strict)"("Val(Sgnl)"=w515) -> ()  [unwired: 2 in, 2 out]
  }
  n221 = call <vilib>:"UeiDaqCloseSession.vi"("error in (no error)"=w4, "UeiDaq Refnum In"=w5) -> ("error out"=w10:errorcluster)  [unwired: 8 in, 1 out]
  n222 = call <vilib>:"UeiDaqShowError.vi"("error in (no error)"=w10) -> ()  [unwired: 10 in, 1 out]
